vi "CRYSet Project Editor Front Panel.vi"(11 "Vi Ref":refnum<vi>) -> ()   [LabVIEW 2013]
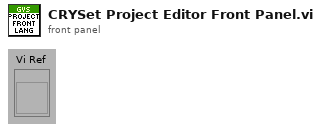
[diagram p1: front panel]
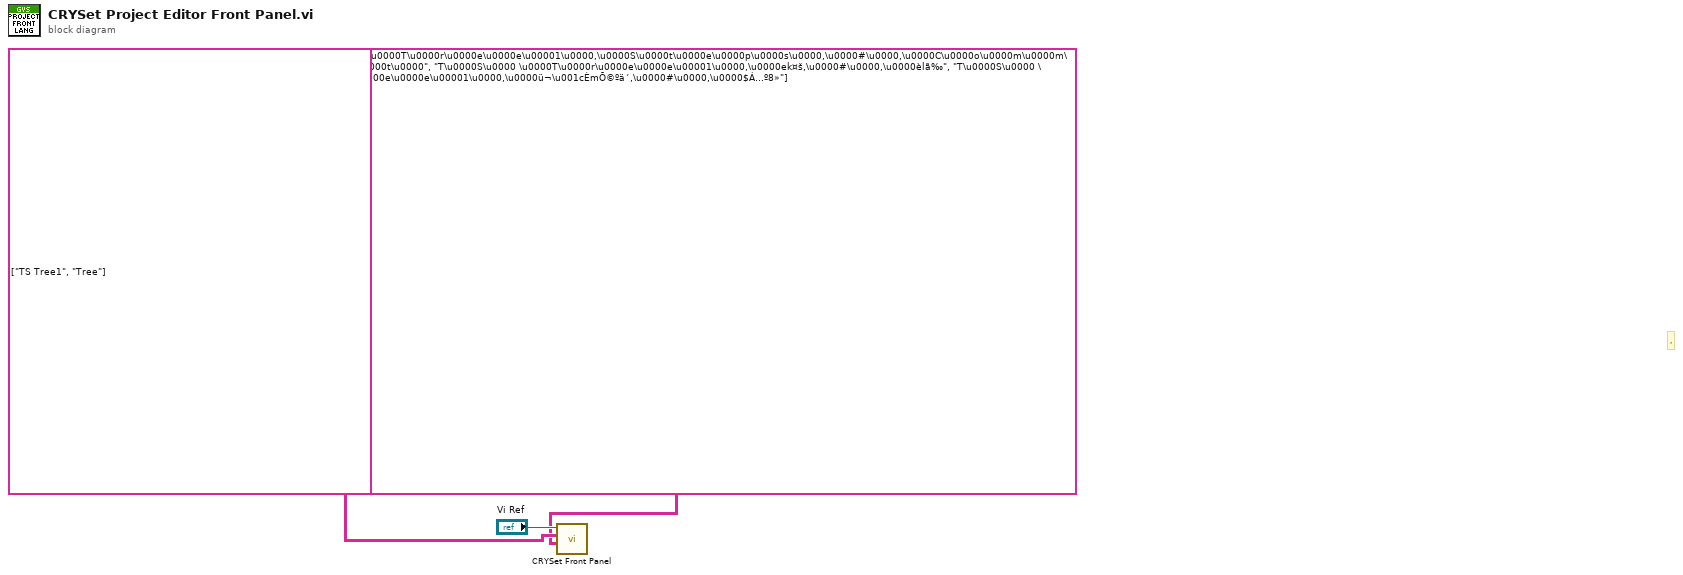
[diagram p0: block diagram]
diagram:
  # ","
  # "Caption, Tab Page, Multilist Header, Button 4"
  # "Control Type"
  # "Control Name and Tab"
  n1 = call "CRYSet Front Panel.vi"("Caption(Boolean Text)"=string[][] [["T\u0000S\u0000 \u0000T\u0000r\u0000e\u0000e\u00001\u0000,\u0000S\u0000t\u0000e\u0000p\u0000s\u0000,\u0000#\u0000,\u0000C\u0000o\u0000m\u0000m\u0000e\u0000n\u0000t\u0000", "T\u0000S\u0000 \u0000T\u0000r\u0000e\u0000e\u00001\u0000,\u0000ek¤š,\u0000#\u0000,\u0000èlã‰", "T\u0000S\u0000 \u0000T\u0000r\u0000e\u0000e\u00001\u0000,\u0000ü¬\u001cÈmÕ©ºä´,\u0000#\u0000,\u0000$Á…º8»"]], "Control ID and Type(Label Name, Type)"=string[][] [["TS Tree1", "Tree"]], "Vi Ref"="Vi Ref") -> ()  [unwired: 9 in]
